vi "Command - Voltage.vi"(0 "VISA Refnum in":refnum<visa-resource-name>, 5 "Channel":i32, 11 "Error In":errorcluster, 12 "Command Type":enum16{"Set", "Get"}(ring)) -> (4 "VISA Refnum out":refnum<visa-resource-name>, 6 "Voltage":string, 8 "Voltage":dbl, 15 "Error Out":errorcluster)   [LabVIEW 2025]
panel:
  in  "Voltage":dbl
  out "return count":u32
  out "Command":string
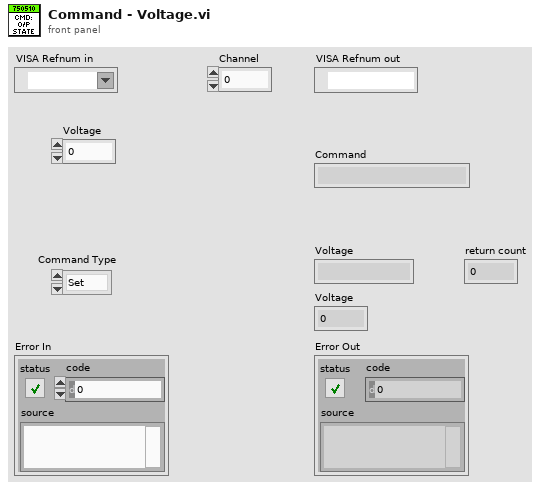
[diagram p1: front panel]
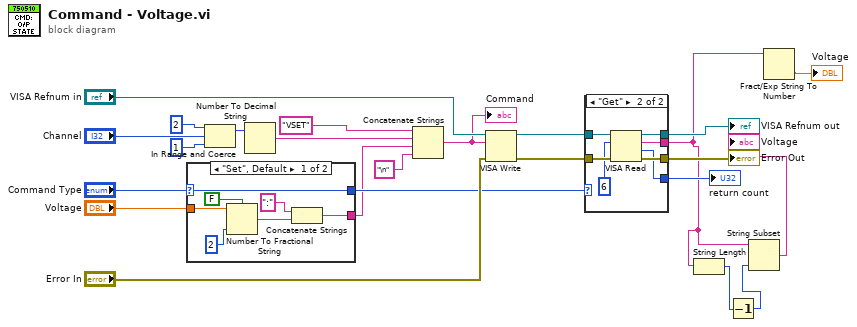
[diagram p0: block diagram]
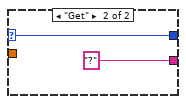
[diagram p2: hidden frame]
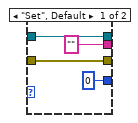
[diagram p3: hidden frame]
diagram:
  n1 = case shown="\"Set\", Default" "Command Type" {
    selector: "Command Type" -> [w31 w32]
    tunnel: [w26 "?" ("string")] -> w7
    tunnel: [w31 w32] -> w10
    tunnel: "Voltage" -> [w30 _]
    frame "Set", Default {
      n2 = Number To Fractional String(use system decimal point (T)=FALSE, number=w30, precision (6)=i16 2 ("width (-)")) -> (F-format string=w27:string)  [unwired: 1 in]
      n3 = Concatenate Strings(":" ("string"), w27) -> (w26:string)
    }
    frame "Get" {
    }
  }
  n4 = In Range and Coerce(upper limit=2, x="Channel", lower limit=1) -> (coerced(x)=w15:i32)  [unwired: 1 out]
  n5 = Number To Decimal String(number=w15) -> (decimal integer string=w17:string)  [unwired: 1 in]
  n6 = Concatenate Strings("VSET", w17, w7, "\n" ("string")) -> (w18:string)
  "Command" <- w18
  n7 = VISA Write(VISA resource name="VISA Refnum in", write buffer=w18, error in (no error)="Error In") -> (VISA resource name out=w20:refnum<visa-resource-name>, error out=w21:errorcluster)  [unwired: 1 out]
  n8 = case shown="\"Get\"" w10 {
    tunnel: w20 -> [w36 w44]
    tunnel: w21 -> [w37 w43]
    tunnel: [w37 w42] -> w22
    tunnel: [w36 w41] -> w23
    tunnel: ["" ("read buffer") w40] -> w2
    tunnel: [u32 0 ("return count") w38] -> w9
    frame "Set", Default {
    }
    frame "Get" {
      n9 = VISA Read(VISA resource name=w44, byte count=u32 6, error in (no error)=w43) -> (VISA resource name out=w41:refnum<visa-resource-name>, read buffer=w40:string, return count=w38:u32, error out=w42:errorcluster)
    }
  }
  "VISA Refnum out" <- w23
  "Error Out" <- w22
  "return count" <- w9
  n10 = String Length(string=w2) -> (length=w4:i32)
  n11 = Decrement(x=w4) -> (x-1=w3:i32)
  n12 = String Subset(string=w2, length (rest)=w3) -> (substring=→"Voltage":string)  [unwired: 1 in]
  n13 = Fract/Exp String To Number(string=w2) -> (number=→"Voltage":dbl)  [unwired: 3 in, 1 out]
